vi "Z900_navX_InternalStartLoop.vi"(8 "error in (no error)":errorcluster, 11 "navX Device":T1={"Interface"={"Protocol"=enum."SERIAL", "Update Rate (4Hz-60Hz)"=4, "navX Open TypeDef"=variant}, "Notify Packet"=refnum, "Loop VI Refnum"=refnum} {"Interface"."Update Rate (4Hz-60Hz)" min=4 max=60 step=1}) -> (0 "error out":errorcluster, 3 "navX Device":T1={"Interface"={"Protocol"=enum."SERIAL", "Update Rate (4Hz-60Hz)"=4, "navX Open TypeDef"=variant}, "Notify Packet"=refnum, "Loop VI Refnum"=refnum} {"Interface"."Update Rate (4Hz-60Hz)" min=4 max=60 step=1})   [LabVIEW 2014, in "navX Library v2.lvlib"]
uses:
  navX Library v2.lvlib
  TypeDefs/Z900_navX_DeviceTypeDef.ctl
  TypeDefs/Z900_navX_ProtocolTypeDef.ctl
  TypeDefs/Z900_navX_NotifyPacketTypeDef.ctl
  TypeDefs/Z900_navX_ActionTypeDef.ctl
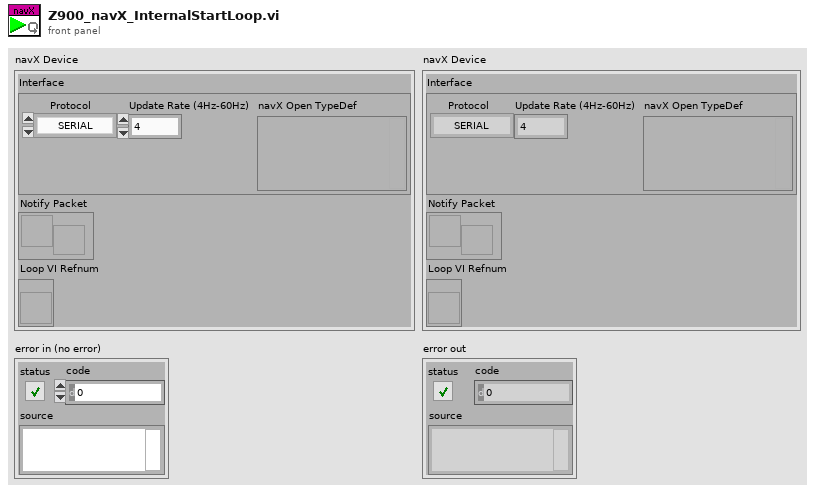
[diagram p1: front panel]
types:
  T1 = typedef "navX Library v2.lvlib/Z900_navX_DeviceTypeDef.ctl" = cluster{"Interface":cluster{"Protocol":T2, "Update Rate (4Hz-60Hz)":u8, "navX Open TypeDef":variant}, "Notify Packet":refnum<notifier>, "Loop VI Refnum":refnum<vi>}
  T2 = typedef "navX Library v2.lvlib/Z900_navX_ProtocolTypeDef.ctl" = enum16{"SERIAL", "I2C", "SPI"}
  T3 = typedef "navX Library v2.lvlib/Z900_navX_NotifyPacketTypeDef.ctl" = cluster{"navX Action":T4, "Data":variant}
  T4 = typedef "navX Library v2.lvlib/Z900_navX_ActionTypeDef.ctl" = enum16{"None", "Halt", "Reboot Detected", "Zero-Yaw"}
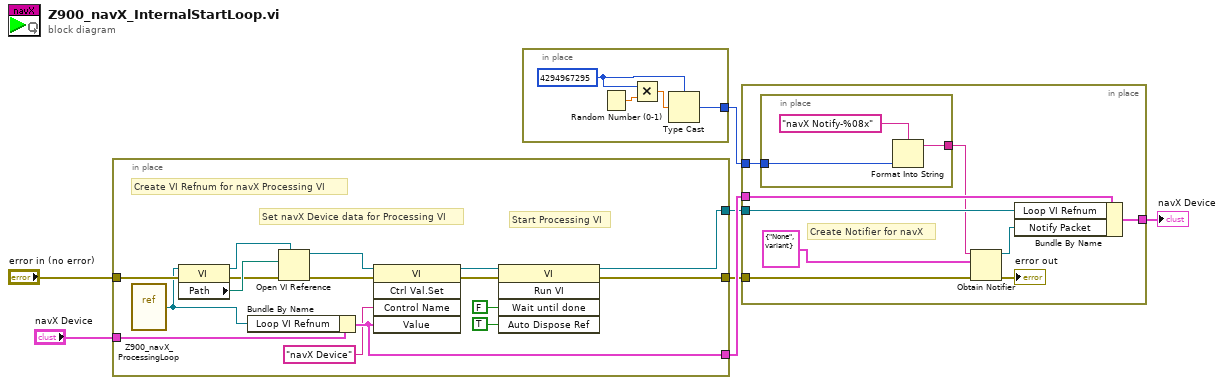
[diagram p0: block diagram]
diagram:
  n1 = in-place {
    in-place-border: "error in (no error)" -> [w23]
    in-place-border: [w13] -> w6
    in-place-border: [w12] -> w5
    in-place-border: [w10] -> w3
    in-place-border: "navX Device" -> [w9]
    # "Start Processing VI"
    # "Set navX Device data for Processing VI"
    # "Create VI Refnum for navX Processing VI"
    n2 = vi-ref "Z900_navX_ProcessingLoop.vi"() -> (w22:refnum<vi>)
    n3 = property class="VI"(reference=w22, error in=w23) -> (reference out=w19:refnum<vi>, error out=w20:errorcluster, "Path"=w21:path)
    n4 = Bundle By Name(cluster=w9, "Loop VI Refnum"=w22) -> (w13:T1)
    n5 = Open VI Reference(type specifier VI Refnum (for type only)=w19, vi path=w21, error in (no error)=w20) -> (vi reference=w11:refnum<vi>, error out=w18:errorcluster)  [unwired: 3 in]
    n6 = invoke class="VI" method="Ctrl Val.Set"(reference=w11, error in=w18, "Control Name"="navX Device" ("format string"), "Value"=w13) -> (reference out=w17:refnum<vi>, error out=w16:errorcluster)  [unwired: 1 in, 3 out]
    n7 = invoke class="VI" method="Run VI"(reference=w17, error in=w16, "Wait until done"=FALSE ("Wait Until Done"), "Auto Dispose Ref"=TRUE ("Auto Dispose Reference")) -> (reference out=w12:refnum<vi>, error out=w10:errorcluster)  [unwired: 1 in, 3 out]
  }
  n8 = in-place {
    in-place-border: [w24] -> w1
    w26 = u32 4294967295
    n9 = Random Number (0-1)() -> (number: 0 to 1=w27:dbl)
    n10 = Multiply(x=w26, y=w27) -> (x*y=w25:dbl)
    n11 = Type Cast(type=w26, x=w25) -> (*(type *) &x=w24:u32)
  }
  n12 = in-place {
    in-place-border: w6 -> [w36]
    in-place-border: w5 -> [w35]
    in-place-border: [w34] -> w4
    in-place-border: w3 -> [w31]
    in-place-border: w1 -> [w28]
    # "Create Notifier for navX"
    n13 = in-place {
      in-place-border: [w38] -> w29
      in-place-border: w28 -> [w37]
      n14 = Format Into String(format string="navX Notify-%08x" ("name (unnamed)"), w37) -> (resulting string=w38:string)  [unwired: 2 in, 1 out]
    }
    n15 = Obtain Notifier(name (unnamed)=w29, notification data type=T3 {"navX Action"=enum."None", "Data"=variant} ("navX Notify Packet"), error in (no error)=w31) -> (notifier out=w33:refnum<notifier>, error out=→"error out":errorcluster)  [unwired: 1 in, 1 out]
    n16 = Bundle By Name(cluster=w36, "Loop VI Refnum"=w35, "Notify Packet"=w33) -> (w34:T1)
  }
  "navX Device" <- w4
